vi "Toggle Selected Edge Annotation Shown.vi"(8 "error in (no error)":errorcluster, 11 "FSM in":refnum<class "FSM.Graph.lvclass">) -> (0 "error out":errorcluster, 3 "FSM out":refnum<class "FSM.Graph.lvclass">)   [LabVIEW 2015, in "FSM.Graph.lvclass"]
uses:
  FSM.Graph.lvclass
  FSM.Graph.lvclass/FSM.Graph.ctl
  FSM.Edge/FSM.Edge.lvclass
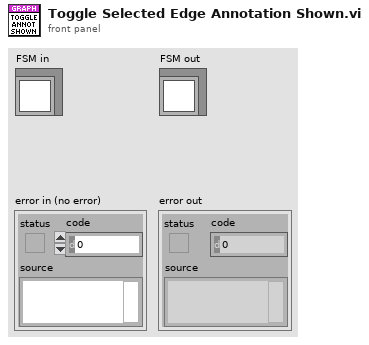
[diagram p1: front panel]
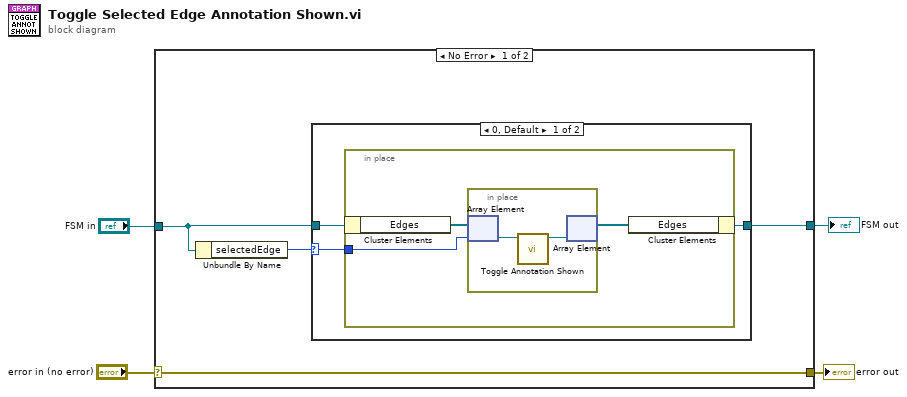
[diagram p0: block diagram]
diagram:
  n1 = case shown="No Error" "error in (no error)" {
    selector: "error in (no error)" -> [w8 w19]
    tunnel: [w8 w19] -> w3
    tunnel: [w5 w18] -> w1
    tunnel: "FSM in" -> [w6 w18]
    frame No Error {
      n2 = Unbundle By Name(w6) -> ("selectedEdge"=w7:i32)
      n3 = case shown="0, Default" w7 {
        selector: w7 -> [w10 _]
        tunnel: w6 -> [w11 w17]
        tunnel: [w9 w17] -> w5
        frame 0, Default {
          n4 = in-place {
            in-place-border: w10 -> [w13]
            n5 = in-place-cluster #1(w11) -> ("Edges"=w14:refnum<class "FSM.Edge.lvclass">[])
            n6 = in-place {
              n7 = in-place-array #2(w14, w13) -> (w16:refnum<class "FSM.Edge.lvclass">)
              n8 = call "Toggle Annotation Shown.vi"("FSM.Edge in"=w16) -> ("FSM.Edge out"=w15:refnum<class "FSM.Edge.lvclass">)  [unwired: 9 in, 1 out]
              n9 = in-place-array #2(w15) -> (w12:refnum<class "FSM.Edge.lvclass">[])  [unwired: 1 out]
            }
            n10 = in-place-cluster #1("Edges"=w12) -> (w9:refnum<class "FSM.Graph.lvclass">)
          }
        }
        frame -1 {
        }
      }
    }
    frame Error {
    }
  }
  "error out" <- w3
  "FSM out" <- w1
